vi "NI 9775 Record Mode 4 channels  (Host).vi"() -> ()   [LabVIEW 2021]
uses:
  <vilib>/LabVIEW Targets/FPGA/cRIO/shared/nicrio_ModuleControls/nicrio_cRIO-9775_TriggerConfigCal.ctl
  <vilib>/LabVIEW Targets/FPGA/cRIO/shared/nicrio_ModuleControls/nicrio_cRIO-9775_TriggerSlope.ctl
  <vilib>/userDefined/High Color/nirio_resource_hc.ctl
  <vilib>/LabVIEW Targets/FPGA/cRIO/shared/nicrio_ModuleControls/nicrio_BasicConversionTime.ctl
  <vilib>/LabVIEW Targets/FPGA/cRIO/shared/nicrio_ModuleControls/nicrio_cRIO-9775_RecordDataRates4ChansRing.ctl
  <vilib>/FPGAPlugInAG/cRIO-9053/niLvFpga_Open_cRIO-9053.vi
  <vilib>/rvi/interface/common/dynamic/niFpgaDynamicAddResources.vi
  <vilib>/FPGAPlugInAG/Dynamic/niLvFpga_Reset_Dynamic.vi
  <vilib>/Utility/error.llb/Error Cluster From Error Code.vi
  <vilib>/rvi/errors/niLvFpgaAdjustHostInterfaceError.vi
  <vilib>/FPGAPlugInAG/Dynamic/niLvFpga_Run_Dynamic.vi
  <vilib>/FPGAPlugInAG/Dynamic/niLvFpga_Close_Dynamic.vi
  <vilib>/rvi/interface/nirviOpenFPGA/nirviOpenFPGA.xnode
  FPGA Bitfiles/ni9775crio9053_FPGATarget2_NI9775GettingSta_5cxlJxftgIw.lvbitx
  NI 9775 Getting Started Record Mode (FPGA).vi
  <vilib>/rvi/interface/nirviMethod/nirviMethod.xnode
  <vilib>/rvi/interface/nirviReadWriteControl/nirviReadWriteControl.xnode
  <vilib>/rvi/interface/nirviCloseFPGA/nirviCloseFPGA.xnode
  <vilib>/rvi/interface/Simulation/niFpgaSimulationCallBeginRW.vi
  <vilib>/FPGAPlugInAG/Dynamic/niLvFpga_ReadFifo_Dynamic.vi
  <vilib>/rvi/errors/niLvFpgaMergeErrorWithErrorCode.vi
  NiFpgaLv.dll
panel:
  in  "Trigger Record Timeout (Ticks)":i32=200000000
  in  "PreTrigger Samples per Record":u32=500
  in  "Samples per Record":u32=1000
  in  "Trigger Type":T1(tab)
  in  "AI Trigger Configuration":T3
  in  "AI 0 Trigger Configuration":T4
  in  "AI 1 Trigger Configuration":T4
  in  "AI 2 Trigger Configuration":T4
  in  "AI 3 Trigger Configuration":T4
  in  "Enable Low Pass Filter":T5
  in  "Fetch Record Timeout (Ticks)":i32=200000000
  out "Fetch Timed Out":bool
  out "Trigger Record Timed Out":bool
  in  "Record Data Rate":T6=1 items=["20.000 MS/s (NI 9775)"=1, "10.00 MS/s (NI 9775)"=2, "6.667 MS/s (NI 9775)"=3, "5.000 MS/s (NI 9775)"=4, "2.500 MS/s (NI 9775)"=8, "1.667 MS/s (NI 9775)"=12, "1.250 MS/s (NI 9775)"=16, "1.000 MS/s (NI 9775)"=20, "833.333 KS/s (NI 9775)"=24, "714.286 KS/s (NI 9775)"=28, "625.000 KS/s (NI 9775)"=32, "555.556 KS/s (NI 9775)"=36, "500.000 KS/s (NI 9775)"=40, "454.545 KS/s (NI 9775)"=44, "416.667 KS/s (NI 9775)"=48, "384.615 KS/s (NI 9775)"=52, "357.143 KS/s (NI 9775)"=56, "333.333 KS/s (NI 9775)"=60, "312.500 KS/s (NI 9775)"=64, "294.118 KS/s (NI 9775)"=68, "277.778 KS/s (NI 9775)"=72, "263.158 KS/s (NI 9775)"=76, "250.000 KS/s (NI 9775)"=80, "238.095 KS/s (NI 9775)"=84, "227.273 KS/s (NI 9775)"=88, "217.391 KS/s (NI 9775)"=92, "208.333 KS/s (NI 9775)"=96, "200.000 KS/s (NI 9775)"=100, "192.308 KS/s (NI 9775)"=104, "185.185 KS/s (NI 9775)"=108, "178.571 KS/s (NI 9775)"=112, "172.414 KS/s (NI 9775)"=116, "166.667 KS/s (NI 9775)"=120, "161.290 KS/s (NI 9775)"=124, "156.250 KS/s (NI 9775)"=128, "151.515 KS/s (NI 9775)"=132, "147.059 KS/s (NI 9775)"=136, "142.857 KS/s (NI 9775)"=140, "138.889 KS/s (NI 9775)"=144, "135.135 KS/s (NI 9775)"=148, "131.579 KS/s (NI 9775)"=152, "128.205 KS/s (NI 9775)"=156, "125.000 KS/s (NI 9775)"=160, "121.951 KS/s (NI 9775)"=164, "119.048 KS/s (NI 9775)"=168, "116.279 KS/s (NI 9775)"=172, "113.636 KS/s (NI 9775)"=176, "111.111 KS/s (NI 9775)"=180, "108.696 KS/s (NI 9775)"=184, "106.383 KS/s (NI 9775)"=188, "104.167 KS/s (NI 9775)"=192, "102.041 KS/s (NI 9775)"=196, "100.000 KS/s (NI 9775)"=200, "50.000 KS/s (NI 9775)"=400, "33.333 KS/s (NI 9775)"=600, "25.000 KS/s (NI 9775)"=800, "20.000 KS/s (NI 9775)"=1000, "16.667 KS/s (NI 9775)"=1200, "14.286 KS/s (NI 9775)"=1400, "12.500 KS/s (NI 9775)"=1600, "11.111 KS/s (NI 9775)"=1800, "10.000 KS/s (NI 9775)"=2000, "9.091 KS/s (NI 9775)"=2200, "8.333 KS/s (NI 9775)"=2400, "7.692 KS/s (NI 9775)"=2600, "7.143 KS/s (NI 9775)"=2800, "6.667 KS/s (NI 9775)"=3000, "6.250 KS/s (NI 9775)"=3200, "5.882 KS/s (NI 9775)"=3400, "5.556 KS/s (NI 9775)"=3600, "5.000 KS/s (NI 9775)"=4000, "4.762 KS/s (NI 9775)"=4200, "4.545 KS/s (NI 9775)"=4400, "4.348 KS/s (NI 9775)"=4600, "4.167 KS/s (NI 9775)"=4800, "4.000 KS/s (NI 9775)"=5000, "3.846 KS/s (NI 9775)"=5200, "3.571 KS/s (NI 9775)"=5600, "3.333 KS/s (NI 9775)"=6000, "3.125 KS/s (NI 9775)"=6400, "2.941 KS/s (NI 9775)"=6800, "2.778 KS/s (NI 9775)"=7200, "2.632 KS/s (NI 9775)"=7600, "2.500 KS/s (NI 9775)"=8000, "2.381 KS/s (NI 9775)"=8400, "2.273 KS/s (NI 9775)"=8800, "2.174 KS/s (NI 9775)"=9200, "2.083 KS/s (NI 9775)"=9600, "2.000 KS/s (NI 9775)"=10000, "1.923 KS/s (NI 9775)"=10400, "1.852 KS/s (NI 9775)"=10800, "1.786 KS/s (NI 9775)"=11200, "1.724 KS/s (NI 9775)"=11600, "1.667 KS/s (NI 9775)"=12000, "1.613 KS/s (NI 9775)"=12400, "1.563 KS/s (NI 9775)"=12800, "1.515 KS/s (NI 9775)"=13200, "1.471 KS/s (NI 9775)"=13600, "1.429 KS/s (NI 9775)"=14000, "1.389 KS/s (NI 9775)"=14400, "1.351 KS/s (NI 9775)"=14800, "1.316 KS/s (NI 9775)"=15200, "1.282 KS/s (NI 9775)"=15600, "1.250 KS/s (NI 9775)"=16000, "1.220 KS/s (NI 9775)"=16400, "1.190 KS/s (NI 9775)"=16800, "1.163 KS/s (NI 9775)"=17200, "1.136 KS/s (NI 9775)"=17600, "1.111 KS/s (NI 9775)"=18000, "1.087 KS/s (NI 9775)"=18400, "1.064 KS/s (NI 9775)"=18800, "1.042 KS/s (NI 9775)"=19200, "1.020 KS/s (NI 9775)"=19600, "1.000 KS/s (NI 9775)"=20000, "0.980 KS/s (NI 9775)"=20400, "0.962 KS/s (NI 9775)"=20800, "0.943 KS/s (NI 9775)"=21200, "0.926 KS/s (NI 9775)"=21600, "0.909 KS/s (NI 9775)"=22000, "0.893 KS/s (NI 9775)"=22400, "0.877 KS/s (NI 9775)"=22800, "0.862 KS/s (NI 9775)"=23200, "0.847 KS/s (NI 9775)"=23600, "0.833 KS/s (NI 9775)"=24000, "0.820 KS/s (NI 9775)"=24400, "0.806 KS/s (NI 9775)"=24800, "0.794 KS/s (NI 9775)"=25200, "0.781 KS/s (NI 9775)"=25600, "0.694 KS/s (NI 9775)"=28800, "0.625 KS/s (NI 9775)"=32000, "0.568 KS/s (NI 9775)"=35200, "0.521 KS/s (NI 9775)"=38400, "0.446 KS/s (NI 9775)"=44800, "0.391 KS/s (NI 9775)"=51200, "0.347 KS/s (NI 9775)"=57600, "0.313 KS/s (NI 9775)"=64000]
  in  "Timing Mode":T7
  out "Host error out":errorcluster
  out "FPGA error out":errorcluster
  out "Waveform Graph":waveform(dbl)[](graph)=[{"t0"=timestamp(0 s since 1904-01-01), "dt"=5e-08, "Y"=array[1000 elements]}, {"t0"=timestamp(0 s since 1904-01-01), "dt"=5e-08, "Y"=array[1000 elements]}, {"t0"=timestamp(0 s since 1904-01-01), "dt"=5e-08, "Y"=array[1000 elements]}, {"t0"=timestamp(0 s since 1904-01-01), "dt"=5e-08, "Y"=array[1000 elements]}]
  out "Elements Remaining":u32
  in  "Host Loop update rate (ms)":u32=100
  in  "RIO Device":T8="RIO0"
  # "Overview: Demonstrates how to acquire record/triggered data from the NI 9775\nRequirements: LabVIEW Full Development System, LV FPGA, and NI RIO\nInstructions: \n1. Configure the Timing, FPGA Input and Trigger Parameters. \n2. Run the VI."
  # "Timing Parameters"
  # "FPGA Input Parameters"
  # "Trigger Parameters"
  # "This tab is intentionally left blank. The FPGA will automatically trigger the NI 9775."
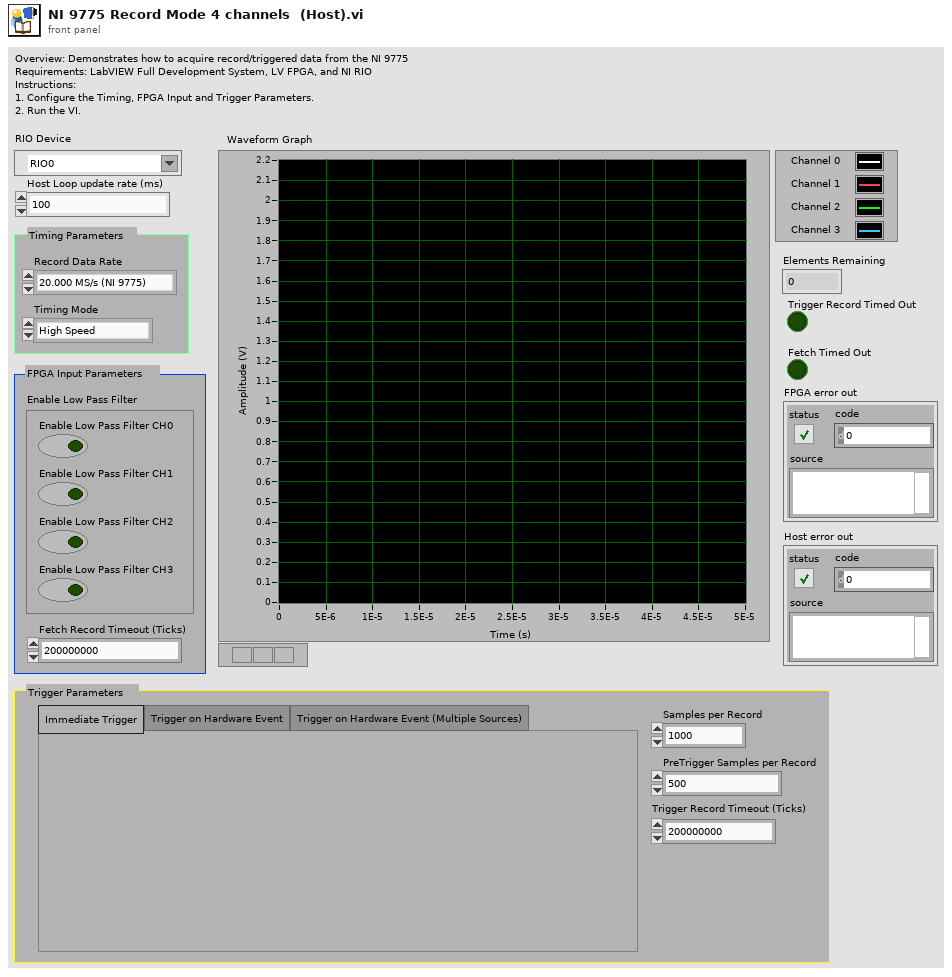
[diagram p1: front panel]
types:
  T1 = enum32{"Immediate Trigger", "Trigger on Hardware Event", "Trigger on Hardware Event (Multiple Sources)"}
  T2 = typedef "nicrio_cRIO-9775_TriggerSlope.ctl" = enum8{"Positive", "Negative"}
  T3 = cluster{"Trigger Slope":T2, "Trigger Level":fxp<+/-,17,5>, "Hystesis Value":fxp<+,16,4>, "AI Channel":u8}
  T4 = typedef "nicrio_cRIO-9775_TriggerConfigCal.ctl" = cluster{"Enable":bool, "Trigger Slope":T2, "Trigger Level":fxp<+/-,17,5>, "Hystesis Value":fxp<+,16,4>}
  T5 = cluster{"Enable Low Pass Filter CH1":bool, "Enable Low Pass Filter CH2":bool, "Enable Low Pass Filter CH3":bool, "Enable Low Pass Filter CH0":bool}
  T6 = typedef "nicrio_cRIO-9775_RecordDataRates4ChansRing.ctl" = u16
  T7 = typedef "nicrio_BasicConversionTime.ctl" = enum8{"High Speed", "High Resolution"}
  T8 = typedef "nirio_resource_hc.ctl" = tag
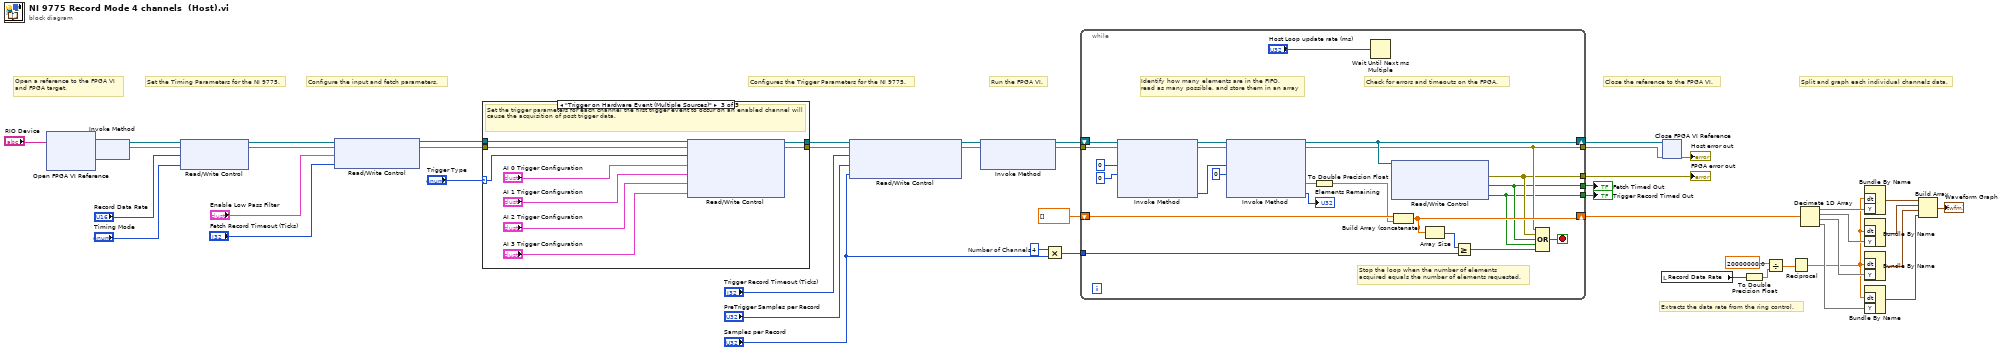
[diagram p0: block diagram]
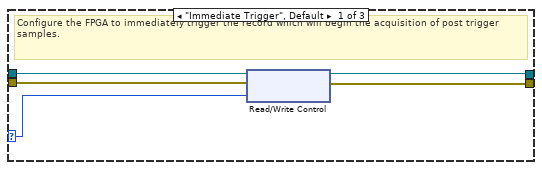
[diagram p2: hidden frame]
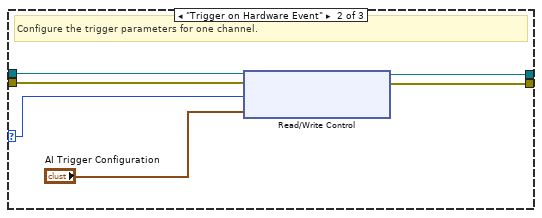
[diagram p3: hidden frame]
diagram:
  w6 = u32 4  # Number of Channels
  # "Configures the Trigger Parameters for the NI 9775."
  # "Configure the input and fetch parameters."
  # "Set the Timing Parameters for the NI 9775."
  # "Split and graph each individual channels data."
  # "Close the reference to the FPGA VI."
  # "Run the FPGA VI."
  # "Open a reference to the FPGA VI \nand FPGA target."
  # "Extracts the data rate from the ring control."
  n1 = xnode "Open FPGA VI Reference"("resource name"="RIO Device") -> ("FPGA VI Reference Out"=w41:refnum<k20>, "error out"=w39:errorcluster)  [unwired: 1 in]
  n2 = xnode "Invoke Method"("FPGA VI Reference In"=w41, "error in"=w39) -> ("FPGA VI Reference Out"=w24:refnum<k20>, "error out"=w23:errorcluster)
  n3 = xnode "Read/Write Control"("FPGA VI Reference In"=w24, "error in"=w23, "Record Data Rate"="Record Data Rate", "Timing Mode"="Timing Mode") -> ("FPGA VI Reference Out"=w20:refnum<k20>, "error out"=w19:errorcluster)
  n4 = xnode "Read/Write Control"("FPGA VI Reference In"=w20, "error in"=w19, "Enable Low Pass Filter"="Enable Low Pass Filter", "Fetch Timeout (Ticks)"="Fetch Record Timeout (Ticks)") -> ("FPGA VI Reference Out"=w18:refnum<k20>, "error out"=w17:errorcluster)
  n5 = case shown="\"Trigger on Hardware Event (Multiple Sources)\"" "Trigger Type" {
    selector: "Trigger Type" -> [w48 w53 w59]
    tunnel: [w50 w58 w67] -> w9
    tunnel: [w51 w57 w66] -> w10
    tunnel: w18 -> [w52 w55 w65]
    tunnel: w17 -> [w49 w56 w64]
    frame "Immediate Trigger", Default {
      # "Configure the FPGA to immediately trigger the record which will begin the acquisition of post trigger samples."
      n6 = xnode "Read/Write Control"("FPGA VI Reference In"=w52, "error in"=w49, "Trigger Type"=w48) -> ("FPGA VI Reference Out"=w51:refnum<k20>, "error out"=w50:errorcluster)
    }
    frame "Trigger on Hardware Event" {
      # "Configure the trigger parameters for one channel."
      n7 = xnode "Read/Write Control"("FPGA VI Reference In"=w55, "error in"=w56, "Trigger Type"=w53, "AI Trigger Configuration"="AI Trigger Configuration") -> ("FPGA VI Reference Out"=w57:refnum<k20>, "error out"=w58:errorcluster)
    }
    frame "Trigger on Hardware Event (Multiple Sources)" {
      # "Set the trigger parameters for each channel the first trigger event to occur on an enabled channel will cause the acquisition of post trigger data."
      n8 = xnode "Read/Write Control"("FPGA VI Reference In"=w65, "error in"=w64, "Trigger Type"=w59, "AI 0 Trigger Configuration"="AI 0 Trigger Configuration", "AI 1 Trigger Configuration"="AI 1 Trigger Configuration", "AI 2 Trigger Configuration"="AI 2 Trigger Configuration", "AI 3 Trigger Configuration"="AI 3 Trigger Configuration") -> ("FPGA VI Reference Out"=w66:refnum<k20>, "error out"=w67:errorcluster)
    }
  }
  n9 = xnode "Read/Write Control"("FPGA VI Reference In"=w10, "error in"=w9, "Trigger Record Timeout (Ticks)"="Trigger Record Timeout (Ticks)", "PreTrigger Samples per Record"="PreTrigger Samples per Record", "Samples per Record"="Samples per Record") -> ("FPGA VI Reference Out"=w11:refnum<k20>, "error out"=w12:errorcluster)
  n10 = xnode "Invoke Method"("FPGA VI Reference In"=w11, "error in"=w12) -> ("FPGA VI Reference Out"=w46:refnum<k20>, "error out"=w47:errorcluster)  [unwired: 1 in]
  n11 = Multiply(x=w6, y="Samples per Record") -> (x*y=w38:u32)
  n12 = while {
    shift-right: [w76] -> w45
    shift-left: w46 -> [w85]
    shift-right: [w78] -> w28
    shift-left: dbl[] [] -> [w80]
    tunnel: w38 -> [w75]
    tunnel: w47 -> [w84]
    tunnel: [w72] -> w44
    tunnel: [w71] -> w40
    tunnel: [w69] -> w25
    tunnel: [w68] -> w26
    stop <- w73 stop-if-true
    # "Check for errors and timeouts on the FPGA."
    # "Stop the loop when the number of elements\nacquired equals the number of elements requested."
    # "Identify how many elements are in the FIFO, \nread as many possible, and store them in an array"
    n13 = xnode "Invoke Method"("FPGA VI Reference In"=w85, "error in"=w84, "Number of Elements"=u32 0, "Timeout (ms)"=0) -> ("FPGA VI Reference Out"=w83:refnum<k20>, "error out"=w82:errorcluster, "Elements Remaining"=w81:u32)  [unwired: 1 out]
    n14 = xnode "Invoke Method"("FPGA VI Reference In"=w83, "error in"=w82, "Number of Elements"=w81, "Timeout (ms)"=0 ("Timeout")) -> ("FPGA VI Reference Out"=w76:refnum<k20>, "error out"=w72:errorcluster, "Data"=w88:fxp<+/-,17,5>[], "Elements Remaining"=→"Elements Remaining":u32)
    n15 = To Double Precision Float(number=w88) -> (double precision float=w79:dbl[])
    n16 = Wait Until Next ms Multiple(millisecond multiple="Host Loop update rate (ms)") -> ()  [unwired: 1 out]
    n17 = xnode "Read/Write Control"("FPGA VI Reference In"=w76) -> ("FPGA Error Out"=w71:errorcluster, "Fetch Timed Out"=w69:bool, "Trigger Record Timed Out"=w68:bool)  [unwired: 1 in, 2 out]
    n18 = Build Array (concatenate)(w80, w79) -> (w78:dbl[])
    n19 = Array Size(array=w78) -> (size(s)=w77:i32)
    n20 = Greater Or Equal?(x=w77, y=w75) -> (x >= y?=w74:bool)
    n21 = Compound Arithmetic op=OR(w72, w71, w69, w68, w74) -> (w73:bool)
  }
  "FPGA error out" <- w40
  "Trigger Record Timed Out" <- w26
  "Fetch Timed Out" <- w25
  n22 = local read "Record Data Rate"() -> (w2:T6)
  n23 = xnode "Close FPGA VI Reference"("FPGA VI Reference In"=w45, "error in"=w44) -> ("error out"=→"Host error out":errorcluster)
  n24 = To Double Precision Float(number=w2) -> (double precision float=w4:dbl)
  n25 = Divide(x=20000000.0, y=w4) -> (x/y=w1:dbl)
  n26 = Reciprocal(x=w1) -> (1/x=w14:dbl)
  n27 = Decimate 1D Array(w28) -> (w37:dbl[], w34:dbl[], w35:dbl[], w30:dbl[])
  n28 = Bundle By Name("dt"=w14, "Y"=w37) -> (w36:waveform(dbl))  [unwired: 1 out]
  n29 = Bundle By Name("dt"=w14, "Y"=w34) -> (w33:waveform(dbl))  [unwired: 1 out]
  n30 = Bundle By Name("dt"=w14, "Y"=w35) -> (w32:waveform(dbl))  [unwired: 1 out]
  n31 = Bundle By Name("dt"=w14, "Y"=w30) -> (w29:waveform(dbl))  [unwired: 1 out]
  n32 = Build Array(w36, w33, w32, w29) -> (→"Waveform Graph":waveform(dbl)[])
